vi "PixelMap_Calculator.vi"(0 "Tot.X.Pixels":u32, 1 "X.Voltage(Max)":dbl, 2 "X.Volt.Offset":dbl, 3 "Tot.Y.Pixels":u32, 4 "Y.Voltage(Max)":dbl, 5 "Y.Volt.Offset":dbl, 6 "X.Pixel.Index":u32, 7 "Y.Pixel.Index":u32) -> (14 "X_Pixel_Voltage":dbl, 16 "Y_Pixel_Voltage":dbl)   [LabVIEW 2012]
uses:
  Custom Controls and Typedefs/Params for Galvo Voltage Calculation (X Axis).ctl
  Custom Controls and Typedefs/Params for Galvo Voltage Calculation (Y Axis).ctl
panel:
  in  "Params for Galvo Voltage Calculation (Y Axis)":T1
  in  "Params for Galvo Voltage Calculation (X Axis)":T2
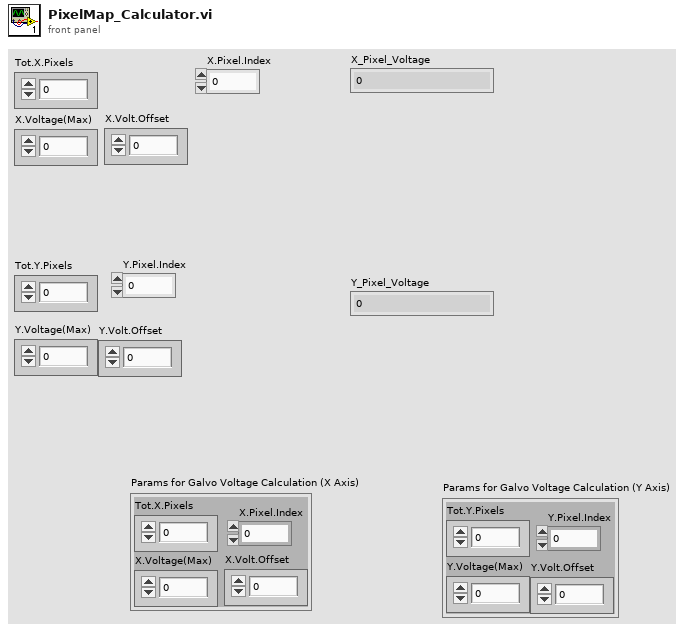
[diagram p1: front panel]
types:
  T1 = typedef "Params for Galvo Voltage Calculation (Y Axis).ctl" = cluster{"Y.Voltage(Max)":dbl, "Y.Volt.Offset":dbl, "Tot.Y.Pixels":u32, "Y.Pixel.Index":u32}
  T2 = typedef "Params for Galvo Voltage Calculation (X Axis).ctl" = cluster{"X.Voltage(Max)":dbl, "X.Volt.Offset":dbl, "Tot.X.Pixels":u32, "X.Pixel.Index":u32}
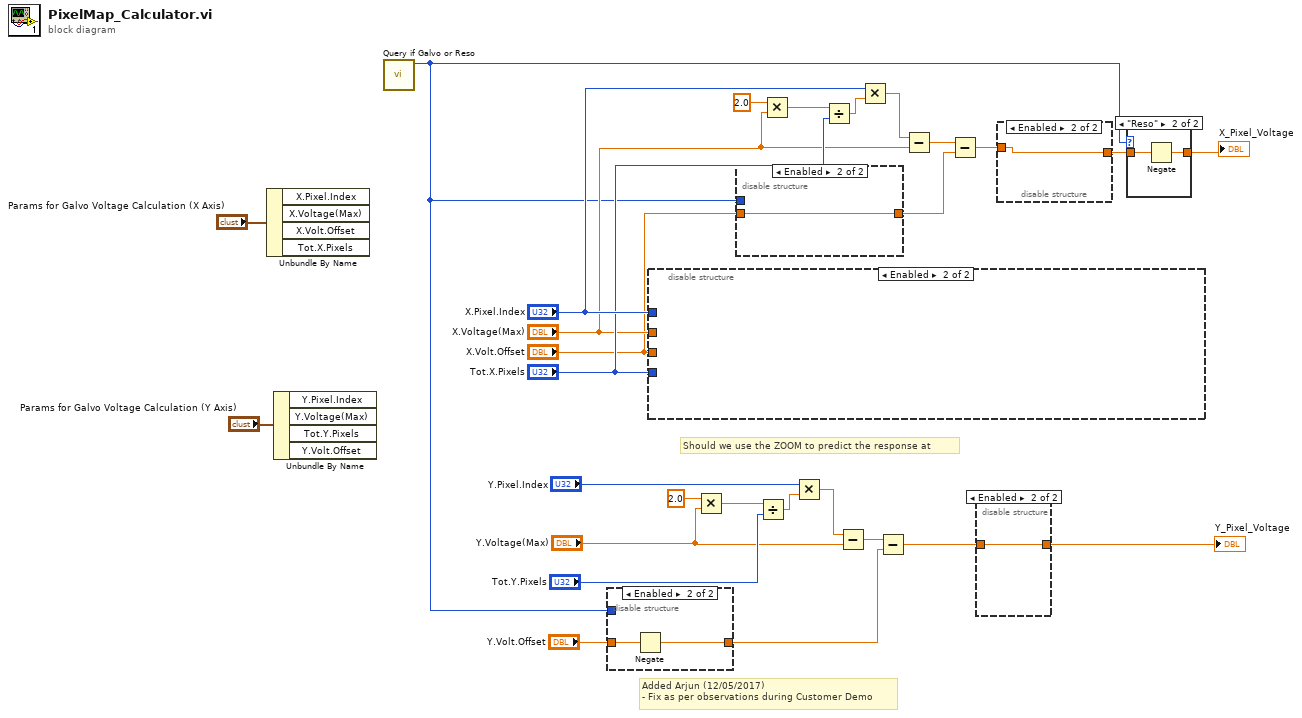
[diagram p0: block diagram]
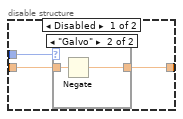
[diagram p2: hidden frame]
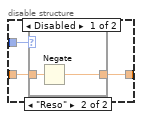
[diagram p4: hidden frame]
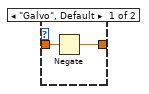
[diagram p6: hidden frame]
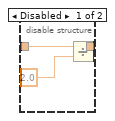
[diagram p7: hidden frame]
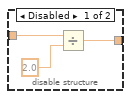
[diagram p8: hidden frame]
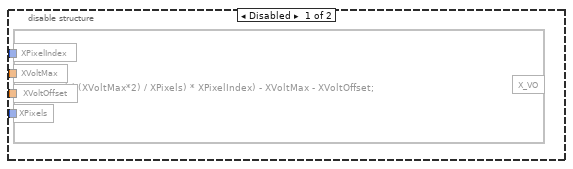
[diagram p9: hidden frame]
diagram:
  # "Added Arjun (12/05/2017)\n- Fix as per observations during Customer Demo"
  # "Should we use the ZOOM to predict the response at"
  n1 = Unbundle By Name("Params for Galvo Voltage Calculation (X Axis)") -> ()  [unwired: 4 out]
  n2 = Unbundle By Name("Params for Galvo Voltage Calculation (Y Axis)") -> ()  [unwired: 4 out]
  n3 = call "Query if Galvo or Reso.vi"() -> ("System Type"=w3:enum16{"Galvo", "Reso"})  [unwired: 10 in, 1 out]
  n4 = disable-structure shown="Enabled" {
    disable-tunnel: "Y.Volt.Offset" -> [w31 w36]
    disable-tunnel: [w30 w35] -> w4
    disable-tunnel: w3 -> [w29 _]
    frame Disabled {
      n5 = case shown="\"Reso\"" w29 {
        tunnel: w31 -> [w32 w34]
        tunnel: [w32 w33] -> w30
        frame "Galvo", Default {
        }
        frame "Reso" {
          n6 = Negate(x=w34) -> (-x=w33:dbl)
        }
      }
    }
    frame Enabled {
      n7 = Negate(x=w36) -> (-x=w35:dbl)
    }
  }
  n8 = disable-structure shown="Enabled" {
    disable-tunnel: "X.Pixel.Index" -> [w40 _]
    disable-tunnel: "X.Voltage(Max)" -> [w39 _]
    disable-tunnel: "Tot.X.Pixels" -> [w38 _]
    disable-tunnel: "X.Volt.Offset" -> [w37 _]
    frame Disabled {
      n9 = formula code="X_VO =  ( ( (XVoltMax*2) / XPixels) * XPixelIndex) - XVoltMax - XVoltOffset;"("XVoltMax"=w39, "XVoltOffset"=w37, "XPixels"=w38, "XPixelIndex"=w40) -> ()  [unwired: 1 out]
    }
    frame Enabled {
    }
  }
  n10 = Multiply(x=2.0, y="Y.Voltage(Max)") -> (x*y=w27:dbl)
  n11 = disable-structure shown="Enabled" {
    disable-tunnel: w3 -> [w43 _]
    disable-tunnel: "X.Volt.Offset" -> [w42 w47]
    disable-tunnel: [w41 w47] -> w1
    frame Disabled {
      n12 = case shown="\"Galvo\"" w43 {
        tunnel: w42 -> [w44 w46]
        tunnel: [w44 w45] -> w41
        frame Default {
        }
        frame "Galvo" {
          n13 = Negate(x=w46) -> (-x=w45:dbl)
        }
      }
    }
    frame Enabled {
    }
  }
  n14 = Divide(x=w27, y="Tot.Y.Pixels") -> (x/y=w22:dbl)
  n15 = Multiply(x=2.0, y="X.Voltage(Max)") -> (x*y=w16:dbl)
  n16 = Multiply(x="Y.Pixel.Index", y=w22) -> (x*y=w20:dbl)
  n17 = Divide(x=w16, y="Tot.X.Pixels") -> (x/y=w18:dbl)
  n18 = Subtract(x=w20, y="Y.Voltage(Max)") -> (x-y=w24:dbl)
  n19 = Multiply(x="X.Pixel.Index", y=w18) -> (x*y=w19:dbl)
  n20 = Subtract(x=w24, y=w4) -> (x-y=w9:dbl)
  n21 = Subtract(x=w19, y="X.Voltage(Max)") -> (x-y=w17:dbl)
  n22 = Subtract(x=w17, y=w1) -> (x-y=w12:dbl)
  n23 = disable-structure shown="Enabled" {
    disable-tunnel: w9 -> [w50 w51]
    disable-tunnel: [w48 w51] -> w10
    frame Disabled {
      n24 = Divide(x=w50, y=2.0) -> (x/y=w48:dbl)
    }
    frame Enabled {
    }
  }
  "Y_Pixel_Voltage" <- w10
  n25 = disable-structure shown="Enabled" {
    disable-tunnel: w12 -> [w54 w55]
    disable-tunnel: [w52 w55] -> w8
    frame Disabled {
      n26 = Divide(x=w54, y=2.0) -> (x/y=w52:dbl)
    }
    frame Enabled {
    }
  }
  n27 = case shown="\"Reso\"" w3 {
    tunnel: w8 -> [w57 w59]
    tunnel: [w56 w58] -> w7
    frame "Galvo", Default {
      n28 = Negate(x=w57) -> (-x=w56:dbl)
    }
    frame "Reso" {
      n29 = Negate(x=w59) -> (-x=w58:dbl)
    }
  }
  "X_Pixel_Voltage" <- w7
